vi "motor control 1.vi"(0 "Tempi":u32[](array[numeric]), 1 "reinitialize? (F)":bool, 2 "1234Speed ref":dbl[](array[numeric])=[0.0, 0.0, 0.0, 0.0], 4 "Automatico (ON)":bool[](array[boolean])=[FALSE, FALSE, FALSE, FALSE], 5 "MANUAL CONTROL":dbl[](array[numeric]), 8 "PID gains":T1(array[cluster])=[{"proportional gain (Kc)"=1.0, "integral time (Ti, min)"=0.01, "derivative time (Td, min)"=0.0}] {"derivative time (Td, min)" format="%.3f"; "integral time (Ti, min)" format="%.3f"; "proportional gain (Kc)" format="%.3f"}, 9 "1234OffSet":dbl[](array[numeric])=[0.0, 0.0, 0.0, 0.0], 11 "1234 Outputs  limits":cluster{"output high":dbl, "output low":dbl}[](array[cluster])=[{"output high"=16000.0, "output low"=-16000.0}, {"output high"=16000.0, "output low"=-16000.0}, {"output high"=16000.0, "output low"=-16000.0}, {"output high"=16000.0, "output low"=-16000.0}]) -> (16 "PWMs":dbl[](array[numeric]), 19 "speeds":dbl[](array[numeric]))   [LabVIEW 2017]
uses:
  <vilib>/addons/control/pid/pid.llb/PID Advanced (DBL Array).vi
  <vilib>/addons/control/pid/pid.llb/PID Parameter Manager (DBL Array).vi
  <vilib>/addons/control/pid/pid.llb/PID Derivative Action Buffered (DBL Array).vi
  <vilib>/addons/control/pid/pid.llb/PID Get Advanced Error (DBL Array).vi
  <vilib>/addons/control/pid/pid.llb/PID Integral Action Buffered (DBL Array).vi
  <vilib>/addons/control/pid/pid.llb/PID Resize 1D Array.vi
  <vilib>/addons/control/pid/pid.llb/PID Get Advanced Error (DBL).vi
  <vilib>/addons/control/pid/pid.llb/PID Advanced (DBL).vi
  <vilib>/addons/control/pid/NI_PID_pid.lvlib
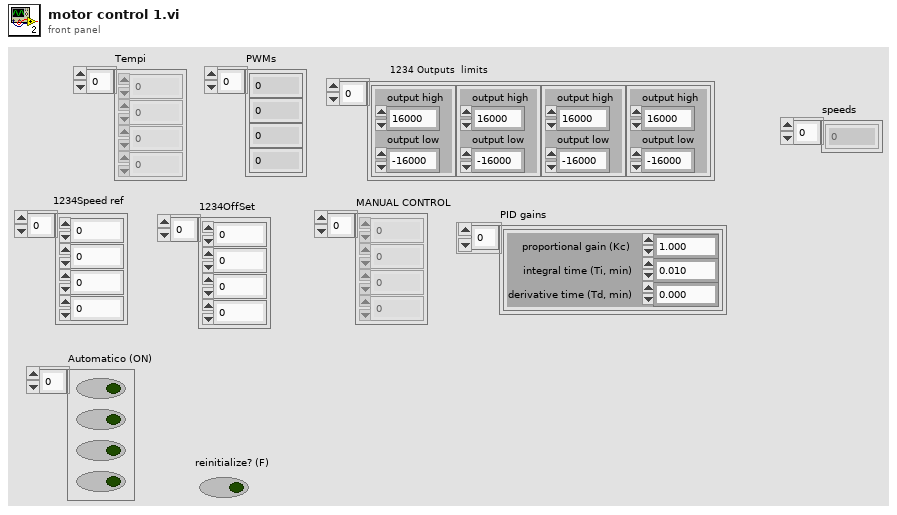
[diagram p1: front panel]
types:
  T1 = cluster{"proportional gain (Kc)":dbl, "integral time (Ti, min)":dbl, "derivative time (Td, min)":dbl}[]
  T2 = cluster{"setpoint high":dbl, "setpoint low":dbl}[]
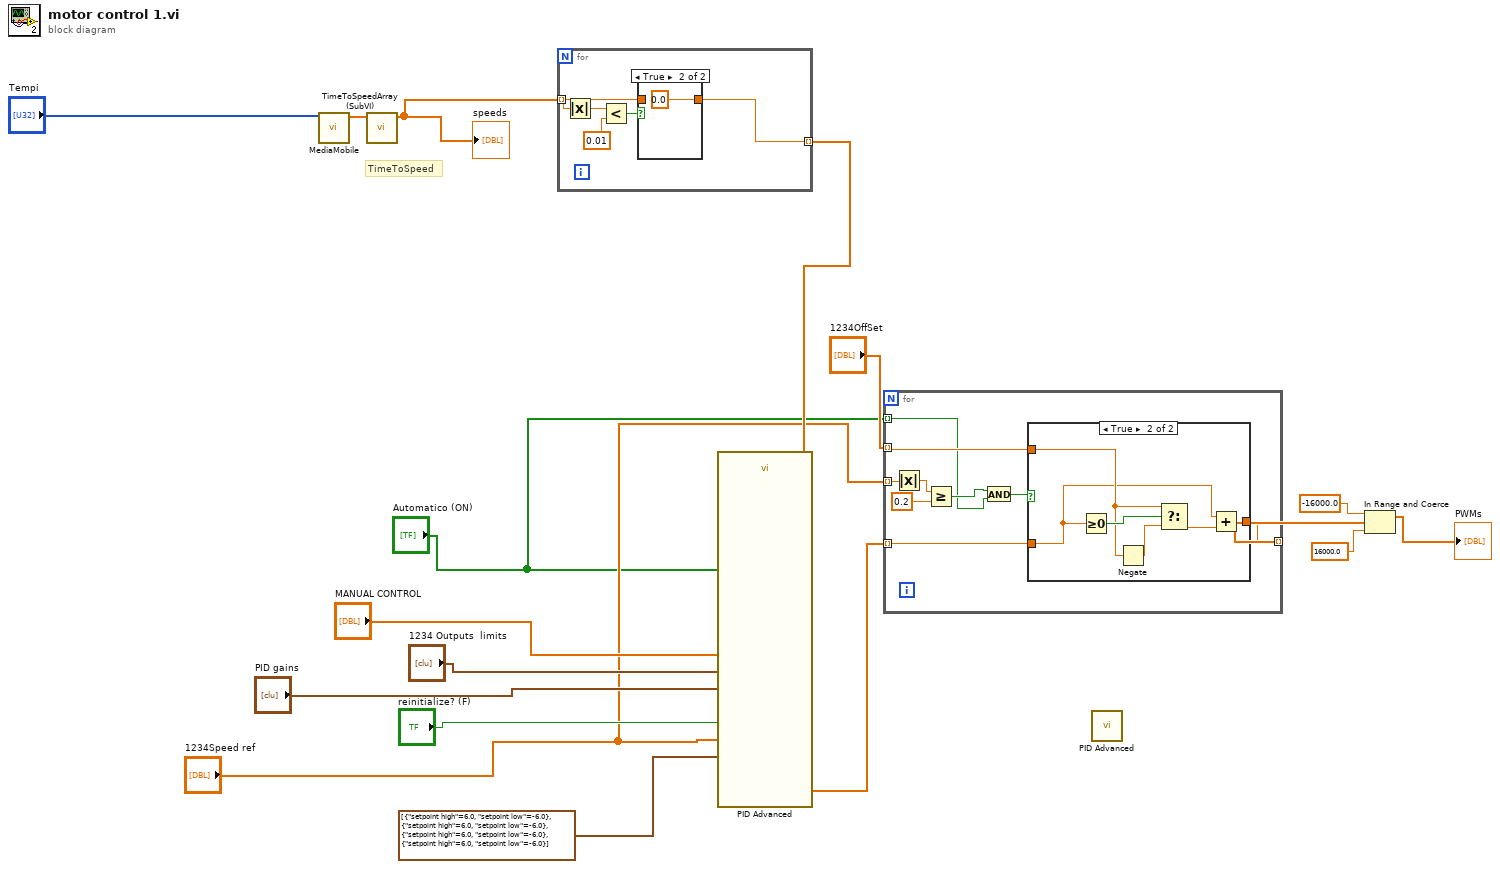
[diagram p0: block diagram]
diagram:
  # "TimeToSpeed"
  n1 = call "MediaMobile.vi"("Tempi Fronti"="Tempi") -> ("Tempi medi"=w17:dbl[])  [unwired: 9 in]
  n2 = call "TimeToSpeedArray (SubVI).vi"("Array"=w17) -> ("Array 2"=w8:dbl[])  [unwired: 10 in]
  "speeds" <- w8
  n3 = for {
    tunnel: w8 -> [w19] mode=indexing
    tunnel: [w20] -> w7 mode=indexing
    n4 = Absolute Value(x=w19) -> (abs(x)=w18:dbl)
    n5 = Less?(x=w18, y=0.01) -> (x < y?=w21:bool)
    n6 = case shown="True" w21 {
      tunnel: [w23 0.0] -> w20
      tunnel: w19 -> [w23 _]
      frame False {
      }
      frame True {
      }
    }
  }
  n7 = call-poly <vilib>:"PID Advanced.vi"("setpoint"="1234Speed ref", "output range"="1234 Outputs  limits", "auto? (T)"="Automatico (ON)", "manual control"="MANUAL CONTROL", "process variable"=w7, "setpoint range"=T2 [{"setpoint high"=6.0, "setpoint low"=-6.0}, {"setpoint high"=6.0, "setpoint low"=-6.0}, {"setpoint high"=6.0, "setpoint low"=-6.0}, {"setpoint high"=6.0, "setpoint low"=-6.0}], "PID gains"="PID gains", "reinitialize? (F)"="reinitialize? (F)") -> ("output"=w10:dbl[])  [unwired: 6 in, 1 out]
  n8 = for {
    tunnel: w10 -> [w32] mode=indexing
    tunnel: [w31] -> w3 mode=indexing
    tunnel: "1234OffSet" -> [w33] mode=indexing
    tunnel: "1234Speed ref" -> [w26] mode=indexing
    tunnel: "Automatico (ON)" -> [w27] mode=indexing
    n9 = Absolute Value(x=w26) -> (abs(x)=w25:dbl)
    n10 = Greater Or Equal?(x=w25, y=0.2) -> (x >= y?=w28:bool)
    n11 = And(x=w28, y=w27) -> (x .and. y?=w29:bool)
    n12 = case shown="True" w29 {
      tunnel: w33 -> [_ w37]
      tunnel: w32 -> [w34 w36]
      tunnel: [w34 w35] -> w31
      frame False {
      }
      frame True {
        n13 = Greater Or Equal To 0?(x=w36) -> (x >= 0?=w40:bool)
        n14 = Negate(x=w37) -> (-x=w39:dbl)
        n15 = Select(t=w37, s=w40, f=w39) -> (s? t:f=w38:dbl)
        n16 = Add(x=w36, y=w38) -> (x+y=w35:dbl)
      }
    }
  }
  n17 = call-poly <vilib>:"PID Advanced.vi"() -> ()  [unwired: 14 in, 2 out]
  n18 = In Range and Coerce(upper limit=-16000.0, x=w3, lower limit=16000.0) -> (coerced(x)=→"PWMs":dbl[])  [unwired: 1 out]
